vi "DTC.StatusCode.Set.vi"(8 "error in":errorcluster, 11 "Section Ref in":T1 format="%.0x") -> (0 "error out":errorcluster, 3 "Section Ref out":T1 format="%.0x")   [LabVIEW 2015, in "Diagnostics Addon System Explorer.lvlib"]
uses:
  Diagnostics Addon System Explorer.lvlib
  <vilib>/NI Veristand/Custom Device API/Custom Device Item Ref.ctl
  Types/FG.Action.ctl
  Shared/SubVIs/Constants.vi
  <vilib>/NI/NI VeriStand Advanced SysDef API/SysDef API/SysDef.Property.Set.vi
  <vilib>/NI/NI VeriStand Advanced SysDef API/_SubVIs/SysDef.Property.Set.I32.vi
  <vilib>/NI/NI VeriStand Advanced SysDef API/_SubVIs/SysDef.Property.Set.U32.vi
  <vilib>/NI/NI VeriStand Advanced SysDef API/_SubVIs/SysDef.Property.Set.DBL.Array.vi
  <vilib>/NI/NI VeriStand Advanced SysDef API/_SubVIs/SysDef.Property.Set.String.Array.vi
  <vilib>/NI Veristand/Custom Device API/NI VeriStand - Get Item Property.vi
  <vilib>/NI Veristand/Custom Device API/Get Item Property (I32).vi
  <vilib>/NI Veristand/Custom Device API/Get Item Property (U32).vi
  <vilib>/NI Veristand/Custom Device API/Get Item Property (Double Array).vi
  <vilib>/NI Veristand/Custom Device API/Get Item Property (String Array).vi
  <vilib>/NI Veristand/Custom Device Tools/Custom Device Utility Library/NI VeriStand - Search for All Items by GUID.vi
  <vilib>/NI Veristand/Custom Device Tools/Custom Device Utility Library/NI VeriStand - Search for Item by Name.vi
  <vilib>/NI VeriStand/Custom Device Tools/Custom Device Utility Library/Custom Device Utility Library.lvlib
  Shared/Diagnostics Addon Shared.lvlib
  <vilib>/NI VeriStand/Custom Device API/Custom Device API.lvlib
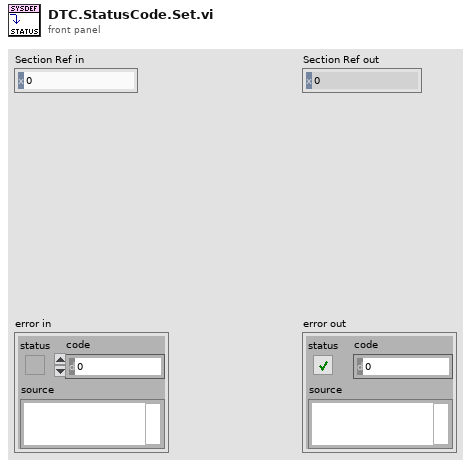
[diagram p1: front panel]
types:
  T1 = typedef "Custom Device API.lvlib/Custom Device Item Ref.ctl" = u64
  T2 = typedef "Diagnostics Addon System Explorer.lvlib/FG.Action.ctl" = enum16{"Get", "Set"}
  T3 = typedef "Diagnostics Addon Shared.lvlib/DTCDescriptor.ctl" = cluster{"DTC Byte Length":i32, "Status Byte Length":i32, "Add Data Byte Length":i32, "Byte Order":enum16{"Motorola", "Intel"}, "DTC.Value.Code":dbl[], "DTC.Value.String":string[], "DTC.Status.Code":dbl[], "DTC.Status.String":string[]}
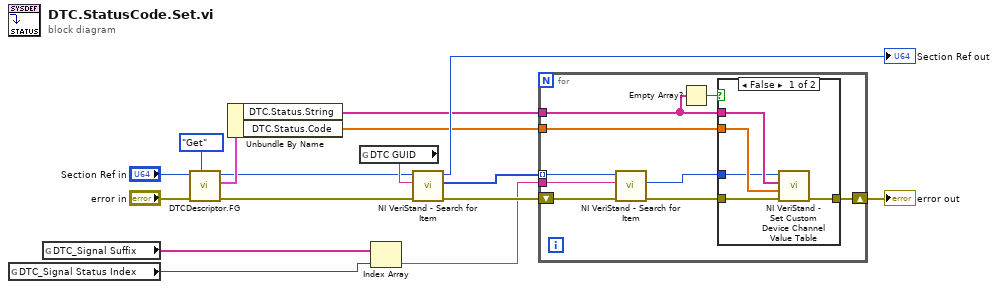
[diagram p0: block diagram]
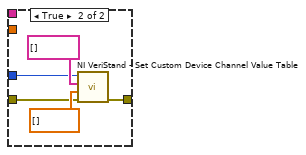
[diagram p2: hidden frame]
diagram:
  n1 = global read "Constants.vi" "DTC_Signal Status Index"() -> (w9:i32)
  n2 = global read "Constants.vi" "DTC_Signal Suffix"() -> (w15:string[])
  n3 = call "DTCDescriptor.FG.vi"("Action"=FG.Action."Get", "error in (no error)"="error in", "Device Item Ref in"="Section Ref in") -> ("error out"=w5:errorcluster, "DTC descriptor"=w7:T3, "Device Item Ref out"=w3:T1)  [unwired: 6 in]
  n4 = Unbundle By Name(w7) -> ("DTC.Status.String"=w1:string[], "DTC.Status.Code"=w2:dbl[])
  n5 = global read "Constants.vi" "DTC GUID"() -> (w16:string)
  n6 = Index Array(array=w15, index=w9) -> (element=w12:string)
  n7 = call-poly <vilib>:"NI VeriStand - Search for Item.vi"("error in"=w5, "Item GUID"=w16, "Section Ref in"=w3) -> ("error out"=w14:errorcluster, "Item Refs"=w13:T1[], "Section Ref out"=→"Section Ref out":T1)  [unwired: 5 in, 1 out]
  n8 = for {
    shift-right: [w19] -> w11
    shift-left: w14 -> [w24]
    tunnel: w13 -> [w23] mode=indexing
    tunnel: w12 -> [w22]
    tunnel: w1 -> [w18]
    tunnel: w2 -> [w17]
    n9 = call-poly <vilib>:"NI VeriStand - Search for Item.vi"("error in"=w24, "Item Name"=w22, "Section Ref in"=w23) -> ("error out"=w20:errorcluster, "Item Ref"=w21:T1)  [unwired: 5 in, 2 out]
    n10 = Empty Array?(array=w18) -> (empty?=w25:bool)
    n11 = case shown="False" w25 {
      tunnel: w18 -> [w30 _]
      tunnel: w17 -> [w29 _]
      tunnel: [w28 w35] -> w19
      tunnel: w21 -> [w26 w32]
      tunnel: w20 -> [w27 w31]
      frame False {
        n12 = call <vilib>:"NI VeriStand - Set Custom Device Channel Value Table.vi"("error in (no error)"=w27, "Values"=w29, "Names"=w30, "Channel Ref in"=w26) -> ("error out"=w28:errorcluster)  [unwired: 6 in, 1 out]
      }
      frame True {
        n13 = call <vilib>:"NI VeriStand - Set Custom Device Channel Value Table.vi"("error in (no error)"=w31, "Values"=dbl[] [], "Names"=string[] [], "Channel Ref in"=w32) -> ("error out"=w35:errorcluster)  [unwired: 6 in, 1 out]
      }
    }
  }
  "error out" <- w11
